vi "pyconnect_0.5.vi"(9 "slider":dbl, 10 "function name":string, 11 "module path":path) -> (3 "Numeric":dbl)   [LabVIEW 2018]
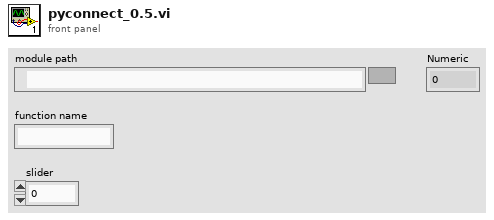
[diagram p1: front panel]
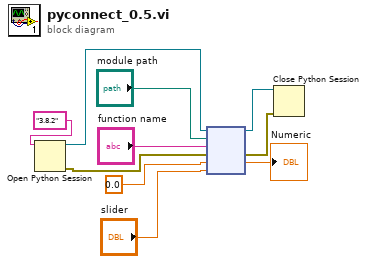
[diagram p0: block diagram]
diagram:
  n1 = Open Python Session(python version="3.8.2" ("Python version")) -> (session out=w7:refnum<k35>, error out=w8:errorcluster)  [unwired: 2 in]
  n2 = node(w7, "module path", "function name", w8, 0.0, "slider") -> (w9:refnum<k35>, w10:errorcluster, →"Numeric":dbl)  [unwired: 1 in, 2 out]
  n3 = Close Python Session(session in=w9, error in=w10) -> ()  [unwired: 1 out]
